vi "Comprar Producto.vi"(8 "error in (no error)":errorcluster, 10 "Comprar":bool, 11 "REFRESCOS Y PAPAS ACTOR in":refnum<class "REFRESCOS Y PAPAS ACTOR.lvclass">) -> (0 "error out":errorcluster, 3 "REFRESCOS Y PAPAS ACTOR out":refnum<class "REFRESCOS Y PAPAS ACTOR.lvclass">)   [LabVIEW 2019, in "REFRESCOS Y PAPAS ACTOR.lvlib" / "REFRESCOS Y PAPAS ACTOR.lvclass"]
uses:
  REFRESCOS Y PAPAS ACTOR.lvclass
  C:/Program Files (x86)/National Instruments/LabVIEW 2019/vi.lib/ActorFramework/Actor/Actor.lvclass
  <vilib>/ActorFramework/Actor/Actor.lvclass/Actor.ctl
  REFRESCOS Y PAPAS ACTOR.lvclass/REFRESCOS Y PAPAS ACTOR.ctl
  UI Actor Messages/Actualizar Estatus Msg/Actualizar Estatus Msg.lvclass/Actualizar Estatus Msg.ctl
  <vilib>/ActorFramework/Message Enqueuer/Message Enqueuer.lvclass/Message Enqueuer.ctl
  UI Actor Messages/Producto Comprado Msg/Producto Comprado Msg.lvclass/Producto Comprado Msg.ctl
  <vilib>/ActorFramework/Message Enqueuer/Enqueue.vi
  UI Actor Messages/Actualizar Estatus Msg/Actualizar Estatus Msg.lvclass
  C:/Program Files (x86)/National Instruments/LabVIEW 2019/vi.lib/ActorFramework/Message/Message.lvclass
  UI Actor Messages/Producto Comprado Msg/Producto Comprado Msg.lvclass
  <vilib>/ActorFramework/Message Priority Queue/Priority Enqueue.vi
  <vilib>/ActorFramework/Actor/Actor.lvclass
panel:
  in  "Cluster Producto":T1
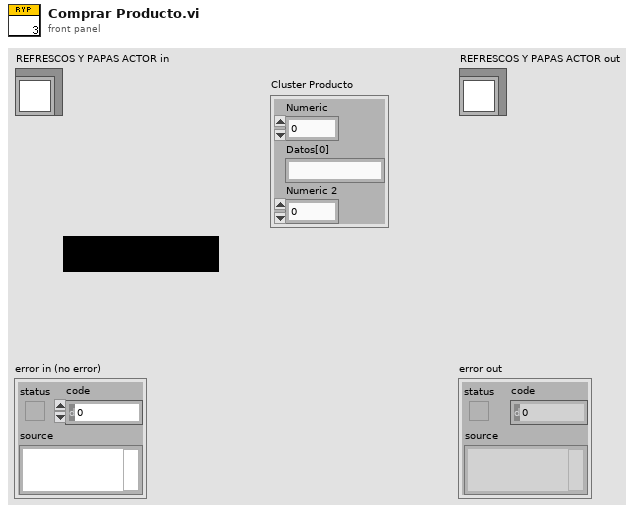
[diagram p1: front panel]
types:
  T1 = cluster{"Numeric":i32, "Datos[0]":string, "Numeric 2":dbl}
  T2 = cluster{"Datos[0]":string, "Datos[1]":string, "Datos[2]":string, "Datos[3]":string, "Datos[4]":string, "Datos[5]":string, "Datos[6]":string, "Datos[7]":string, "Datos[8]":string}
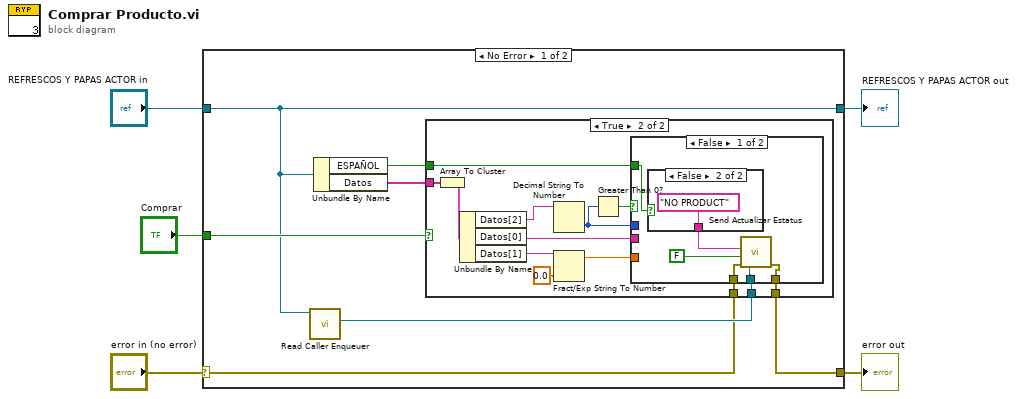
[diagram p0: block diagram]
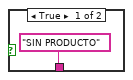
[diagram p3: hidden frame]
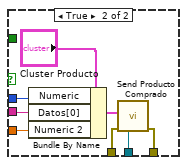
[diagram p4: hidden frame]
diagram:
  n1 = case shown="No Error" "error in (no error)" {
    selector: "error in (no error)" -> [w8 w44]
    tunnel: [w7 w44] -> w4
    tunnel: [w10 w43] -> w2
    tunnel: "REFRESCOS Y PAPAS ACTOR in" -> [w10 w43]
    tunnel: "Comprar" -> [w11 _]
    frame No Error {
      n2 = call <vilib>:"Read Caller Enqueuer.vi"("Actor"=w10) -> ("Caller Enqueuer"=w9:refnum<class "Message Enqueuer.lvclass">)  [unwired: 10 in]
      n3 = Unbundle By Name(w10) -> ("ESPAÑOL"=w6:bool, "Datos"=w12:string[])
      n4 = case shown="True" w11 {
        tunnel: w12 -> [_ w20]
        tunnel: w9 -> [_ w17]
        tunnel: w8 -> [w13 w16]
        tunnel: [w13 w15] -> w7
        tunnel: w6 -> [_ w14]
        frame False {
        }
        frame True {
          n5 = Array To Cluster(array=w20) -> (cluster=w26:T2)
          n6 = Unbundle By Name(w26) -> ("Datos[2]"=w19:string, "Datos[0]"=w24:string, "Datos[1]"=w18:string)
          n7 = Decimal String To Number(string=w19) -> (number=w21:i32)  [unwired: 2 in, 1 out]
          n8 = Fract/Exp String To Number(string=w18, default (0 dbl)=0.0 ("default (0 I32)")) -> (number=w23:dbl)  [unwired: 2 in, 1 out]
          n9 = Greater Than 0?(x=w21) -> (x > 0?=w22:bool)
          n10 = case shown="False" w22 {
            tunnel: w24 -> [_ w40]
            tunnel: w23 -> [_ w39]
            tunnel: w21 -> [_ w41]
            tunnel: w17 -> [w29 w37]
            tunnel: w16 -> [w31 w36]
            tunnel: [w30 w35] -> w15
            tunnel: w14 -> [w32 _]
            frame False {
              n11 = case shown="False" w32 {
                tunnel: ["SIN PRODUCTO" ("Message") "NO PRODUCT" ("Message")] -> w28
                frame True {
                }
                frame False {
                }
              }
              n12 = call "Send Actualizar Estatus.vi"("error in (no error)"=w31, "ACTUALIZA TABLA"=FALSE, "ESTATUS"=w28, "Message Enqueuer"=w29) -> ("error out"=w30:errorcluster)  [unwired: 6 in, 1 out]
            }
            frame True {
              n13 = Bundle By Name(cluster="Cluster Producto", "Numeric"=w41, "Datos[0]"=w40, "Numeric 2"=w39) -> (w38:T1)
              n14 = call "Send Producto Comprado.vi"("error in (no error)"=w36, "Cluster Producto"=w38, "Message Enqueuer"=w37) -> ("error out"=w35:errorcluster)  [unwired: 7 in, 1 out]
            }
          }
        }
      }
    }
    frame Error {
    }
  }
  "error out" <- w4
  "REFRESCOS Y PAPAS ACTOR out" <- w2
